vi "SVFA Zoom FFT Spectrum (Real-Im) (N Ch).vi"(0 "scaled signals [EU]":waveform(dbl)[](array[waveform]), 3 "zoom settings":T2={"frequency range"={"start frequency"=1000.0, "stop frequency"=2000.0}, "window"=1, "number of lines"=400, "% overlap"=0.0} {"% overlap" min=0.0 format="%.2f"; "number of lines" min=2; "window" items=["None ", "Hanning", "Hamming", "Blackman-Harris", "Exact Blackman", "Blackman", "Flat Top", "4 Term B-Harris ", "7 Term B-Harris", "Low Sidelobe"]; "frequency range"."stop frequency" min=0.0 format="%.2f"; "frequency range"."start frequency" min=0.0 format="%.2f"}, 5 "error in (no error)":errorcluster, 7 "averaging parameters":T9={"averaging mode"=enum."No averaging", "weighting mode"=enum."Exponential", "number of averages"=10, "linear mode"=enum."One shot"} {"number of averages" min=1 step=1}, 9 "restart averaging (F)":bool) -> (11 "averaging done":bool, 12 "new spectrum available":bool, 13 "averages completed":dbl, 14 "real parts [EU rms]":cluster{"f0":dbl, "df":dbl, "real part":dbl[]}[](array[cluster]) {"real part" format="%.2p"; "df" format="%.2p"; "f0" format="%.2p"}, 16 "imaginary parts [EU rms]":T1(array[cluster]) {"imaginary part" format="%.2p"; "df" format="%.2p"; "f0" format="%.2p"}, 17 "unit labels":string[](array[string]), 18 "spectrum info":T3[](array[typedef]) {"x-axis units" items=["Time (s)"=0, "Frequency-CB (Hz)"=1, "Frequency-CPB (Hz)"=1248, "Frequency-Arbitrary (Hz)"=2357, "Quefrency (s)"=2, "Revolutions (rev)"=3, "Order"=4, "Speed (RPM)"=11, "Speed (rad/s)"=21, "Index"=65535]; "weighting filter" items=["Linear", "A-weighting", "B-weighting", "C-weighting", "ITU-R 468-4", "Dolby", "CCITT", "C-message", "Wb", "Wc", "Wd", "We", "Wf", "Wh", "Wj", "Wk", "Wm", "AES17 20 kHz lowpass", "AES17 40 kHz lowpass", "AES17 20 kHz highpass", "AES17 40 kHz highpass"]; "dB reference [EU]" format="%.2f"; "engineering units" items=["custom..."=0, "V"=1, "A"=21, "C"=30, "pC"=31, "s"=32, "-"=29, "Pa"=2, "N"=20, "g"=3, "m/s^2"=4, "m/s"=5, "m"=6, "mm/s"=12, "mm"=13, "micron/s"=14, "micron"=15, "in/s^2"=7, "in/s"=8, "in"=9, "mil/s"=10, "mil"=11, "rad/s^2"=16, "rad/s"=17, "rad"=18, "deg/s^2"=26, "deg/s"=27, "deg"=28, "RPM"=22, "cycle/s^2"=23, "Hz"=24, "cycle"=25, "strain"=19]; "spectral info"."window" items=["None "=0, "Hanning"=1, "Hamming"=2, "Blackman-Harris"=3, "Exact Blackman"=4, "Blackman"=5, "Flat Top"=6, "4 Term B-Harris "=7, "7 Term B-Harris"=8, "Low Sidelobe"=9, "Force - Exponential"=10, "Gaussian"=62]}, 19 "error out":errorcluster)   [LabVIEW 2017]
doc: "Computes the zoom FFT spectrum of <B>scaled signal [EU]</B> and <B>zoom settings</B>. Zoom FFT results are returned as real part and imaginary part. Data accumulates each time this VI is called. However, it returns a new spectrum only when sufficient data accumulates. Indicators and subsequent processing should only be called when <B>new spectrum available</B> is TRUE. Wire data to the <B>scaled signal [EU]</B> input to determine the polymorphic instance to use or manually select the instance."
uses:
  <vilib>/addons/_NISVFA/_Shared subVIs/Controls/svc_Spectrum Info.ctl
  <vilib>/addons/_NISVFA/_Shared subVIs/Controls/svc_X-Axis Units.ctl
  <vilib>/addons/_NISVFA/_Shared subVIs/Controls/svc_Spectrum Type.ctl
  <vilib>/addons/_NISVFA/_Shared subVIs/Controls/svc_Engineering Units Text Ring.ctl
  <vilib>/addons/_NISVFA/_Shared subVIs/Controls/svc_Weighting Filter Text Ring.ctl
  <vilib>/addons/_NISVFA/_Shared subVIs/Controls/svc_Complimentary Spectrum Units.ctl
  <vilib>/addons/_NISVFA/_Shared subVIs/Spectrum Info/svfa_Build Spectrum Info.vi
  <vilib>/addons/_NISVFA/_Shared subVIs/Spectrum Averaging/svfa_Reset Averaging State Info.vi
  <vilib>/addons/_NISVFA/_Shared subVIs/Spectrum Averaging/svfa_Average Array with Avg Checks (complex) No State.vi
  <vilib>/addons/_NISVFA/_Shared subVIs/Common/svc_Complex to Mag2 Array.vi
  <vilib>/addons/_NISVFA/_Shared subVIs/Spectrum Averaging/svfa_Average Array with Avg Checks (real) No State.vi
  <vilib>/addons/_NISVFA/_Shared subVIs/Common/svc_Get SV Channel Info.vi
  <vilib>/addons/_NISVFA/_Shared subVIs/Common/svc_Spectrum Units.vi
  <vilib>/addons/_NISVFA/_Shared subVIs/Spectrum Averaging/svfa_Average Array (complex) No State.vi
  <vilib>/addons/_NISVFA/_Shared subVIs/Spectrum Averaging/svfa_Average Array (real) No State.vi
  <vilib>/addons/_NISVFA/_Shared subVIs/Spectrum Averaging/svfa_No Average Array (complex).vi
  <vilib>/addons/_NISVFA/_Shared subVIs/Spectrum Averaging/svfa_Average Array (complex).vi
  <vilib>/addons/_NISVFA/_Shared subVIs/Spectrum Averaging/svfa_No Average Array (real).vi
  <vilib>/addons/_NISVFA/_Shared subVIs/Spectrum Averaging/svfa_Average Array (real).vi
  <vilib>/addons/_NISVFA/_Shared subVIs/Spectrum Averaging/svfa_Peak Hold Array.vi
  <vilib>/addons/_NISVFA/_Shared subVIs/Common/svc_Get Weighting Enum and Labels.vi
  <vilib>/addons/_NISVFA/_Shared subVIs/Common/svc_Unit Label Lexical Class.vi
  <vilib>/addons/_NISVFA/_Shared subVIs/Common/svc_Engineering Units to Unit Label.vi
  <vilib>/addons/_NISVFA/_Shared subVIs/Common/svc_Format Value (DBL).vi
  <vilib>/addons/_NISVFA/_Shared subVIs/Common/svc_Channel Info to Spectrum Info.vi
  <vilib>/addons/_NISVFA/_Shared subVIs/Common/svc_Unit Label to Engineering Units.vi
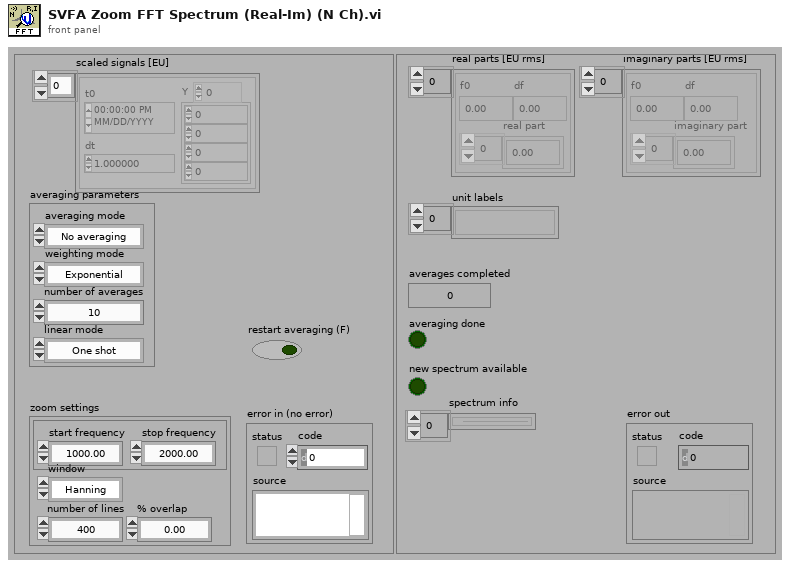
[diagram p1: front panel]
types:
  T1 = cluster{"f0":dbl, "df":dbl, "imaginary part":dbl[]}[]
  T2 = cluster{"frequency range":cluster{"start frequency":dbl, "stop frequency":dbl}, "window":u16, "number of lines":i32, "% overlap":dbl}
  T3 = typedef "svc_Spectrum Info.ctl" = cluster{"channel name":string, "description":string, "x-axis units":T4, "spectral info":cluster{"spectrum type":T5, "linear/dB":enum16{"linear", "dB"}, "window":u16, "window size":i32, "FFT size":i32}, "engineering units":T6, "custom label":string, "dB reference [EU]":dbl, "peak units":enum16{"rms", "peak", "peak-peak"}, "weighting filter":T7, "spectral density?":bool, "unit label":string, "spectrum skewed?":bool, "complimentary spectrum units":T8}
  T4 = typedef "svc_X-Axis Units.ctl" = u16
  T5 = typedef "svc_Spectrum Type.ctl" = enum16{"FFT Spectrum [complex]", "Amplitude [Magnitude]", "Power [Magnitude^2]", "Cross Spectrum [complex]", "Frequency Response [Complex]"}
  T6 = typedef "svc_Engineering Units Text Ring.ctl" = u16
  T7 = typedef "svc_Weighting Filter Text Ring.ctl" = u16
  T8 = typedef "svc_Complimentary Spectrum Units.ctl" = enum16{"none", "radians", "degrees", "cycles", "imaginary"}
  T9 = cluster{"averaging mode":enum16{"No averaging", "Vector averaging", "RMS averaging", "Peak hold"}, "weighting mode":enum16{"Linear", "Exponential"}, "number of averages":u32, "linear mode":enum16{"One shot", "Auto restart"}}
  T10 = enum16{"Restart processing", "Continue processing", "Skip processing"}
  T11 = enum16{"No averaging", "Vector averaging", "RMS averaging", "Peak hold"}
  T12 = cluster{"f0":dbl, "df":dbl, "complex FFT":cdb[]}[]
  T13 = cluster{"zoom settings":cluster{"center frequency":dbl, "zoom":i32, "trim":dbl}, "FFT settings":cluster{"window":enum16{"None ", "Hanning", "Hamming", "Blackman-Harris", "Exact Blackman", "Blackman", "Flat Top", "4 Term B-Harris ", "7 Term B-Harris", "Low Sidelobe"}, "window size":i32, "FFT size":i32, "%overlap":dbl}}
  T14 = cluster{"complex FFT":cdb[], "real FFT":dbl[], "f0":dbl, "df":dbl, "averages completed":dbl, "averaging parameters":cluster{"averaging mode":enum16{"No averaging", "Vector averaging", "RMS averaging", "Peak hold"}, "weighting mode":enum16{"Linear", "Exponential"}, "number of averages":u32, "linear mode":enum16{"One shot", "Auto restart"}}}[]
  T15 = cluster{"complex FFT":cdb[], "real FFT":dbl[], "f0":dbl, "df":dbl, "averages completed":dbl, "averaging parameters":cluster{"averaging mode":enum16{"No averaging", "Vector averaging", "RMS averaging", "Peak hold"}, "weighting mode":enum16{"Linear", "Exponential"}, "number of averages":u32, "linear mode":enum16{"One shot", "Auto restart"}}}
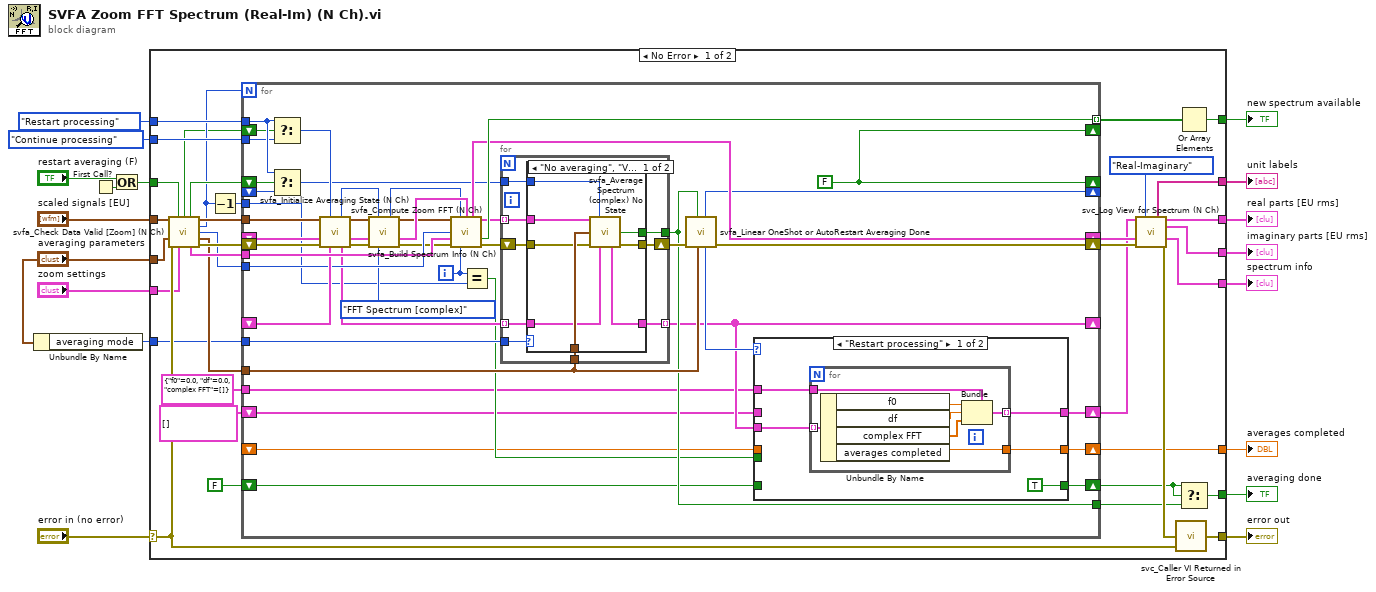
[diagram p0: block diagram]
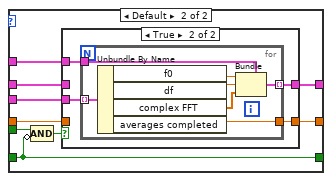
[diagram p2: hidden frame]
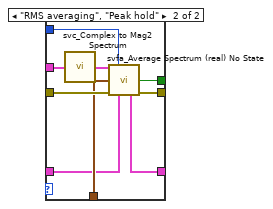
[diagram p4: hidden frame]
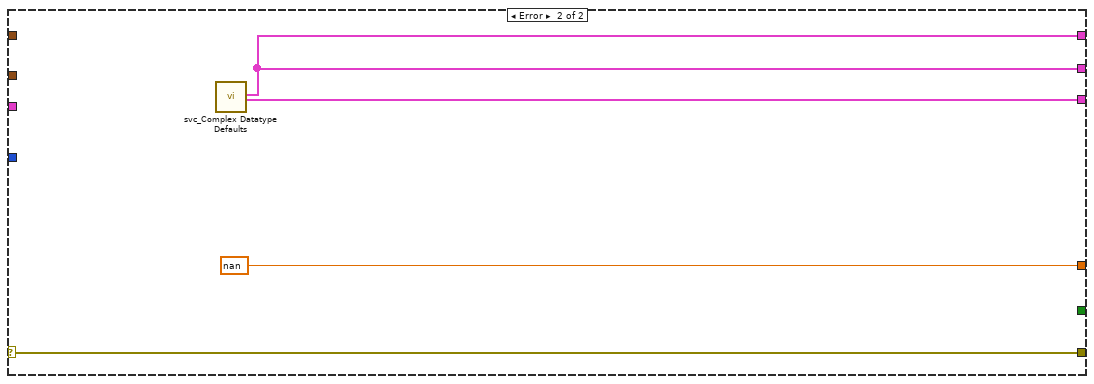
[diagram p5: hidden frame]
diagram:
  n1 = Unbundle By Name("averaging parameters") -> ("averaging mode"=w3:T11)
  n2 = First Call?() -> (First Call?: T/F=w7:bool)
  n3 = Or(x="restart averaging (F)", y=w7) -> (x .or. y?=w5:bool)
  n4 = case shown="No Error" "error in (no error)" {
    selector: "error in (no error)" -> [w46 w163]
    tunnel: w5 -> [w33 _]
    tunnel: [w21 nan ("Averaged So-far")] -> w9
    tunnel: "averaging parameters" -> [w52 _]
    tunnel: "zoom settings" -> [w44 _]
    tunnel: "scaled signals [EU]" -> [w54 _]
    tunnel: [w48 w160] -> w10
    tunnel: [w53 _] -> w13
    tunnel: [w50 w161] -> w8
    tunnel: [w51 w161] -> w12
    tunnel: [w34 _] -> w14
    tunnel: [w47 w163] -> w11
    tunnel: [w24 _] -> w18
    tunnel: w3 -> [w32 _]
    tunnel: T10."Restart processing" ("processing control in") -> [w31 _]
    tunnel: T10."Continue processing" ("processing control in") -> [w30 _]
    frame No Error {
      n5 = call <vilib>:"svfa_Check Data Valid [Zoom] (N Ch).vi"("scaled signals [EU]"=w54, "restart averaging (F)"=w33, "averaging parameters"=w52, "error in (no error)"=w46, "zoom settings"=w44) -> ("reset processing"=w27:bool, "restart averaging"=w36:bool, "dup scaled signals"=w43:waveform(dbl)[], "iterations"=w29:i32, "maximum block size"=w35:i32, "dup averaging parameters"=w40:T9, "zoom FFT settings"=w41:T13, "error out"=w42:errorcluster)  [unwired: 3 in]
      n6 = Decrement(x=w29) -> (x-1=w28:i32)
      n7 = for {
        N: w29 -> [_]
        shift-left: _ -> [w94]
        shift-right: [w60] -> _
        tunnel: [w95] -> w38 mode=indexing
        tunnel: w41 -> [w97]
        tunnel: w43 -> [w98]
        tunnel: [w67] -> w23
        tunnel: w40 -> [w91]
        shift-right: [w93] -> w37
        shift-left: _ -> [w92]
        shift-right: [w64] -> _
        shift-left: _ -> [w90]
        tunnel: w31 -> [w73]
        tunnel: w35 -> [w88]
        shift-right: [w65] -> _
        shift-left: w36 -> [w89]
        shift-right: [w99] -> w39
        shift-left: w42 -> [w96]
        tunnel: w32 -> [w74]
        tunnel: w30 -> [w72]
        tunnel: w28 -> [w69]
        shift-right: [w65] -> _
        shift-left: w27 -> [w66]
        shift-right: [w58] -> w20
        shift-left: T12 [] -> [w57]
        shift-right: [w56] -> w21
        shift-left: _ -> [w55]
        shift-right: [w62] -> w25
        shift-left: FALSE ("restart averaging") -> [w61]
        tunnel: cluster{"f0":dbl, "df":dbl, "complex FFT":cdb[]} {"f0"=0.0, "df"=0.0, "complex FFT"=[]} -> [w59]
        i -> [w68]
        w65 = FALSE ("restart averaging")
        n8 = Select(t=w73, s=w66, f=w72) -> (s? t:f=w71:T10)
        n9 = Select(t=w73, s=w89, f=w90) -> (s? t:f=w70:T10)
        n10 = call <vilib>:"svfa_Initialize Averaging State (N Ch).vi"("Windowed Waveform(s)"=w98, "processing control in"=w71, "spectra info in"=w92, "error in (no error)"=w96, "state info"=w94) -> ("processing control out"=w79:T10, "Windowed Waveform(s)"=w81:waveform(dbl)[], "spectra info out"=w80:T3[], "state info"=w77:T14, "error out"=w82:errorcluster)  [unwired: 6 in]
        n11 = call <vilib>:"svfa_Build Spectrum Info (N Ch).vi"("scaled signal(s)"=w81, "processing control in"=w79, "spectra info in"=w80, "error in (no error)"=w82, "spectrum type"=svc_Spectrum_Type."FFT Spectrum [complex]") -> ("dup processing control"=w76:T10, "dup scaled signals"=w78:waveform(dbl)[], "spectra info out"=w86:T3[], "error out"=w75:errorcluster)  [unwired: 7 in]
        n12 = call <vilib>:"svfa_Compute Zoom FFT (N Ch).vi"("scaled signals [EU]"=w78, "processing control"=w76, "spectra info in"=w86, "maximum block size"=w88, "zoom FFT settings"=w97, "error in (no error)"=w75, "iteration"=w68) -> ("spectra info out"=w93:T3[], "FFT spectra"=w84:cluster{"f0":dbl, "df":dbl, "spectrum":cdb[]}[], "spectrum ready"=w95:bool, "error out"=w83:errorcluster)  [unwired: 4 in, 1 out]
        n13 = Equal?(x=w68, y=w69) -> (x = y?=w63:bool)
        n14 = for {
          tunnel: w91 -> [w142]
          tunnel: w74 -> [w141]
          tunnel: [w139] -> w67
          tunnel: [w138] -> w60 mode=indexing
          tunnel: w84 -> [w137] mode=indexing
          tunnel: w70 -> [w135]
          tunnel: w77 -> [w134] mode=indexing
          shift-right: [w140] -> w87
          shift-left: w83 -> [w136]
          n15 = case shown="\"No averaging\", \"Vector averaging\"" w141 {
            tunnel: w142 -> [w149 w157]
            tunnel: [w147 w153] -> w140
            tunnel: [w146 w158] -> w139
            tunnel: w137 -> [w150 w154]
            tunnel: w136 -> [w148 w159]
            tunnel: w135 -> [w145 w155]
            tunnel: [w144 w151] -> w138
            tunnel: w134 -> [w143 w152]
            frame "No averaging", "Vector averaging" {
              n16 = call <vilib>:"svfa_Average Spectrum (complex) No State.vi"("spectrum"=w150, "processing control"=w145, "averaging parameters"=w149, "error in (no error)"=w148, "averaging state info in"=w143) -> ("averaging done"=w146:bool, "averaging state info out"=w144:T15, "error out"=w147:errorcluster)  [unwired: 5 in, 3 out]
            }
            frame "RMS averaging", "Peak hold" {
              n17 = call <vilib>:"svc_Complex to Mag2 Spectrum.vi"("complex spectrum"=w154) -> ("power spectrum"=w156:cluster{"f0":dbl, "df":dbl, "spectrum":dbl[]})  [unwired: 4 in]
              n18 = call <vilib>:"svfa_Average Spectrum (real) No State.vi"("spectrum"=w156, "processing control"=w155, "averaging parameters"=w157, "error in (no error)"=w159, "averaging state info in"=w152) -> ("averaging done"=w158:bool, "averaging state info out"=w151:T15, "error out"=w153:errorcluster)  [unwired: 5 in, 3 out]
            }
          }
        }
        n19 = call <vilib>:"svfa_Linear OneShot or AutoRestart Averaging Done.vi"("averaging parameters"=w91, "averaging done"=w67, "error in (no error)"=w87) -> ("error out"=w99:errorcluster, "processing control"=w64:T10)  [unwired: 7 in]
        n20 = case shown="\"Restart processing\"" w64 {
          tunnel: w60 -> [w104 w120]
          tunnel: [TRUE ("restart averaging") w115] -> w62
          tunnel: [w102 w119] -> w58
          tunnel: w61 -> [_ w115]
          tunnel: w63 -> [_ w118]
          tunnel: w59 -> [w101 w117]
          tunnel: [w100 w114] -> w56
          tunnel: w55 -> [_ w113]
          tunnel: w57 -> [_ w112]
          frame "Restart processing" {
            n21 = for {
              tunnel: w104 -> [w108] mode=indexing
              tunnel: [w107] -> w102 mode=indexing
              tunnel: w101 -> [w106]
              tunnel: [w105] -> w100
              n22 = Unbundle By Name(w108) -> ("f0"=w111:dbl, "df"=w110:dbl, "complex FFT"=w109:cdb[], "averages completed"=w105:dbl)
              n23 = Bundle(cluster=w106, "f0"=w111, "df"=w110, "complex FFT"=w109) -> (w107:cluster{"f0":dbl, "df":dbl, "complex FFT":cdb[]})
            }
          }
          frame Default {
            n24 = Compound Arithmetic op=AND(w118, invert w115) -> (w116:bool)
            n25 = case shown="True" w116 {
              tunnel: w120 -> [_ w126]
              tunnel: [w121 w125] -> w119
              tunnel: w117 -> [_ w124]
              tunnel: [w122 w123] -> w114
              tunnel: w113 -> [w122 _]
              tunnel: w112 -> [w121 _]
              frame False {
              }
              frame True {
                n26 = for {
                  tunnel: w126 -> [w130] mode=indexing
                  tunnel: [w129] -> w125 mode=indexing
                  tunnel: w124 -> [w128]
                  tunnel: [w127] -> w123
                  n27 = Unbundle By Name(w130) -> ("f0"=w133:dbl, "df"=w132:dbl, "complex FFT"=w131:cdb[], "averages completed"=w127:dbl)
                  n28 = Bundle(cluster=w128, "f0"=w133, "df"=w132, "complex FFT"=w131) -> (w129:cluster{"f0":dbl, "df":dbl, "complex FFT":cdb[]})
                }
              }
            }
          }
        }
      }
      n29 = call <vilib>:"svc_Log View for Spectrum (N Ch).vi"("complex spectra"=w20, "View"=enum16{"Mag-Phase", "Real-Imaginary"}."Real-Imaginary", "spectra info in"=w37, "error in (no error)"=w39) -> ("unit label [mag or real]"=w53:string[], "magnitude or real"=w51:cluster{"f0":dbl, "df":dbl, "magnitude":dbl[]}[], "phase or imaginary"=w50:cluster{"f0":dbl, "df":dbl, "magnitude":dbl[]}[], "spectra info out"=w48:T3[], "error out"=w49:errorcluster)  [unwired: 6 in, 1 out]
      n30 = call <vilib>:"svc_Caller VI Returned in Error Source.vi"("warning input to caller"=w46, "error in (no error)"=w49) -> ("error out"=w47:errorcluster)  [unwired: 3 in]
      n31 = Or Array Elements(Boolean array=w38) -> (logical OR=w34:bool)
      n32 = Select(t=w25, s=w25, f=w23) -> (s? t:f=w24:bool)
    }
    frame Error {
      n33 = call <vilib>:"svc_Complex Datatype Defaults.vi"() -> ("empty array of spectra"=w161:cluster{"f0":dbl, "df":dbl, "magnitude":dbl[]}[], "empty array of spectrum info"=w160:T3[])  [unwired: 11 in, 7 out]
    }
  }
  "averages completed" <- w9
  "new spectrum available" <- w14
  "error out" <- w11
  "spectrum info" <- w10
  "unit labels" <- w13
  "real parts [EU rms]" <- w12
  "imaginary parts [EU rms]" <- w8
  "averaging done" <- w18
